vi "Set Velocity Setpoint.vi"(8 "error in (no error)":errorcluster, 10 "CCW velocity (rad/s)":dbl, 11 "KUKA youBot wheel motor_EtherCAT in":refnum<class "NI_Robotics_KUKA youBot Wheel Motor_EtherCAT.lvclass">) -> (0 "error out":errorcluster, 3 "KUKA youBot wheel motor_EtherCAT out":refnum<class "NI_Robotics_KUKA youBot Wheel Motor_EtherCAT.lvclass">)   [LabVIEW 2017, in "NI_Robotics_KUKA youBot Host.lvlib" / "NI_Robotics_KUKA youBot Wheel Motor_EtherCAT.lvclass"]
uses:
  <vilib>/robotics/KUKA youBot/Motor/Wheel Motor EtherCAT/NI_Robotics_KUKA youBot Wheel Motor_EtherCAT.lvclass
  <vilib>/robotics/KUKA youBot/Motor/Wheel Motor EtherCAT/NI_Robotics_KUKA youBot Wheel Motor_EtherCAT.lvclass/NI_Robotics_KUKA youBot Wheel Motor_EtherCAT.ctl
  <vilib>/robotics/KUKA youBot/NI_Robotics_KUKA youBot Host.lvlib
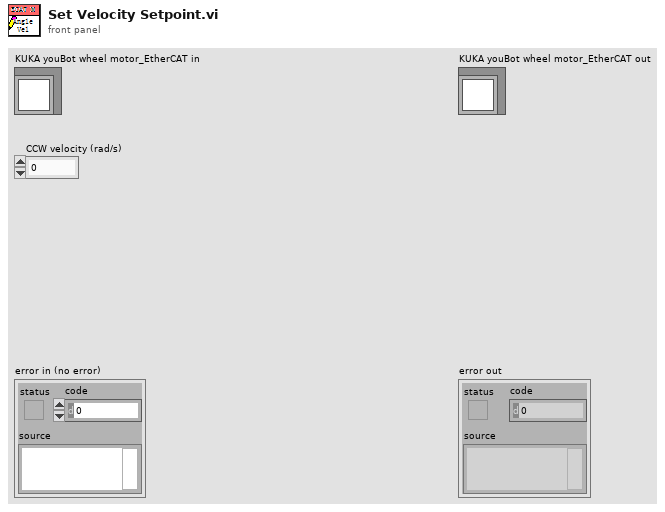
[diagram p1: front panel]
types:
  T1 = typedef "NI_Robotics_KUKA youBot Host.lvlib/Motor Slave Info.ctl" = cluster{"controller mode var":refnum<k21>, "reference var":refnum<k21>, "current var":refnum<k21>, "velocity var":refnum<k21>, "position var":refnum<k21>, "status var":refnum<k21>, "valid":bool, "status var type":enum16{"Int16", "Int32"}, "nodeAddr":u16, "masterHdl":T2}
  T2 = typedef "NI_Robotics_KUKA youBot Host.lvlib/Mater Handler.ctl" = i32
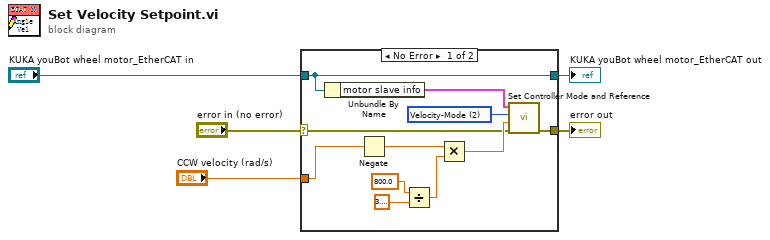
[diagram p0: block diagram]
diagram:
  n1 = case shown="No Error" "error in (no error)" {
    selector: "error in (no error)" -> [w6 w17]
    tunnel: "CCW velocity (rad/s)" -> [w8 _]
    tunnel: "KUKA youBot wheel motor_EtherCAT in" -> [w13 w18]
    tunnel: [w16 w17] -> w1
    tunnel: [w13 w18] -> w2
    frame No Error {
      w14 = u8 2 items=["Motor Stop", "Positioning-Mode", "Velocity-Mode", "no more action", "set position to reference", "PWM-Mode", "Current-Mode", "Initialize"] ("controller mode")
      n2 = Unbundle By Name(w13) -> ("motor slave info"=w15:T1)
      n3 = Negate(x=w8) -> (-x=w9:dbl)
      n4 = Divide(x=800.0 ("y"), y=3.141592653589793) -> (x/y=w10:dbl)
      n5 = Multiply(x=w9, y=w10) -> (x*y=w7:dbl)
      n6 = call <vilib>:"Set Controller Mode and Reference.vi"("error in (no error)"=w6, "reference"=w7, "controller mode"=w14, "motor slave info in"=w15) -> ("error out"=w16:errorcluster)  [unwired: 5 in, 2 out]
    }
    frame Error {
    }
  }
  "error out" <- w1
  "KUKA youBot wheel motor_EtherCAT out" <- w2
